vi "current_vi_path_stripped2.vi"(4 "current VI Path":path) -> (1 "exe?":bool, 2 "current VI Path stripped out":path)   [LabVIEW 2017]
doc: "Input is \"current VI Path\". Depending on whether the path is called from inside an exe or VI, the path is being stripped twice or ones. Therefore, output is the path to folder of the \"current VI\""
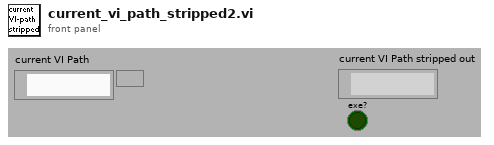
[diagram p1: front panel]
types:
  T1 = enum32{"invalid app kind", "Development System", "Run Time System", "Student Edition", "Embedded LabVIEW", "Evaluation", "Custom"}
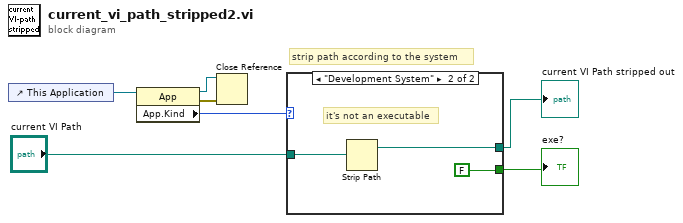
[diagram p0: block diagram]
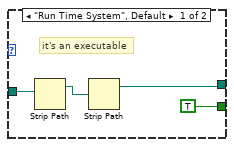
[diagram p2: hidden frame]
diagram:
  # "strip path according to the system"
  n1 = control-ref of="This Application"() -> (w7:refnum<vi>)
  n2 = property class="App"(reference=w7) -> (reference out=w5:refnum<vi>, error out=w6:errorcluster, "App.Kind"=w4:T1)  [unwired: 1 in]
  n3 = Close Reference(reference=w5, error in (no error)=w6) -> ()  [unwired: 1 out]
  n4 = case shown="\"Development System\"" w4 {
    tunnel: "current VI Path" -> [w11 w14]
    tunnel: [w9 w13] -> w1
    tunnel: [TRUE FALSE] -> w2
    frame "Run Time System", Default {
      # "it's an executable"
      n5 = Strip Path(path=w11) -> (stripped path=w10:path)  [unwired: 1 out]
      n6 = Strip Path(path=w10) -> (stripped path=w9:path)  [unwired: 1 out]
    }
    frame "Development System" {
      # "it's not an executable"
      n7 = Strip Path(path=w14) -> (stripped path=w13:path)  [unwired: 1 out]
    }
  }
  "current VI Path stripped out" <- w1
  "exe?" <- w2
